vi "DAC Run.vi"(8 "error in":errorcluster, 11 "DAC Traverse in":refnum<class "DAC Traverse.lvclass">) -> (0 "error out":errorcluster, 3 "DAC Traverse out":refnum<class "DAC Traverse.lvclass">)   [LabVIEW 2019, in "DAC.lvlib" / "DAC Traverse.lvclass"]
uses:
  DAC Traverse.lvclass
  C:/Users/krio/Documents/LV_Projects/test-stand/App/DAC/DAC.lvclass
  DAC.lvclass/DAC.ctl
  Results/Results Method.ctl
  Results/Water Tunnel Results/Water Tunnel Results.lvclass
  DAC Traverse.lvclass/DAC Traverse.ctl
  DAC.lvclass
  Results/Results.lvlib
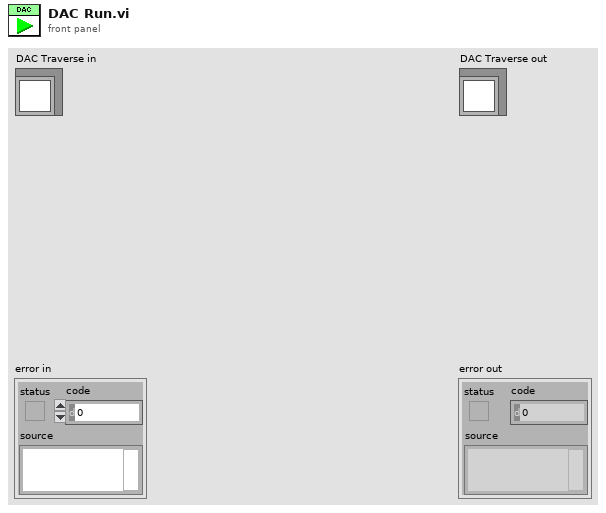
[diagram p1: front panel]
types:
  T1 = typedef "Results.lvlib/Results Method.ctl" = enum16{"Get", "Set"}
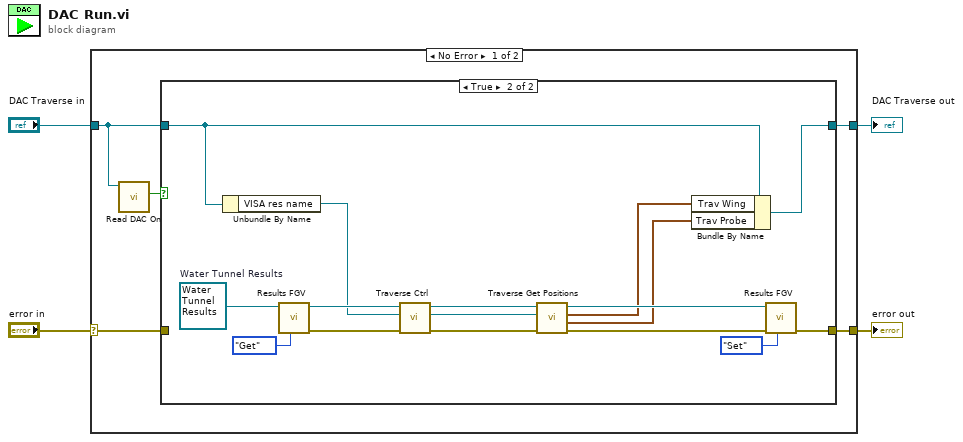
[diagram p0: block diagram]
diagram:
  n1 = case shown="No Error" "error in" {
    selector: "error in" -> [w7 w29]
    tunnel: [w6 w29] -> w2
    tunnel: [w8 w28] -> w1
    tunnel: "DAC Traverse in" -> [w5 w28]
    frame No Error {
      n2 = call "Read DAC On.vi"("DAC in"=w5) -> ("DAC On"=w9:bool)  [unwired: 8 in, 2 out]
      n3 = case shown="True" w9 {
        tunnel: w5 -> [w11 w27]
        tunnel: [w11 w24] -> w8
        tunnel: w7 -> [w10 _]
        tunnel: [w10 w23] -> w6
        frame False {
        }
        frame True {
          w22 = refnum<class "Water Tunnel Results.lvclass"> refnum  # Water Tunnel Results
          n4 = Unbundle By Name(w27) -> ("VISA res name"=w19:refnum<visa-resource-name>)
          n5 = call-dynamic "Results FGV.vi"("Method"=Results_Method."Get", "Water Tunnel Results in"=w22) -> ("error out"=w20:errorcluster, "Water Tunnel  Results out"=w21:refnum<class "Water Tunnel Results.lvclass">)  [unwired: 8 in]
          n6 = call "Traverse Ctrl.vi"("error in"=w20, "VISA resource name"=w19, "Water Tunnel Results in"=w21) -> ("error out"=w17:errorcluster, "VISA resource name out"=w12:refnum<visa-resource-name>, "Water Tunnel Results out"=w18:refnum<class "Water Tunnel Results.lvclass">)  [unwired: 6 in]
          n7 = call "Traverse Get Positions.vi"("error in"=w17, "VISA resource name"=w12, "Water Tunnel Results in"=w18) -> ("error out"=w16:errorcluster, "Trav Probe"=w13:cluster{"Px":dbl, "Py":dbl, "Pz":dbl}, "Trav Wing"=w14:cluster{"Wx":dbl, "Wy":dbl, "Wz":dbl}, "Water Tunnel Results out"=w15:refnum<class "Water Tunnel Results.lvclass">)  [unwired: 5 in]
          n8 = Bundle By Name(cluster=w27, "Trav Wing"=w14, "Trav Probe"=w13) -> (w24:refnum<class "DAC Traverse.lvclass">)
          n9 = call-dynamic "Results FGV.vi"("Method"=Results_Method."Set", "error in"=w16, "Water Tunnel Results in"=w15) -> ("error out"=w23:errorcluster)  [unwired: 7 in, 1 out]
        }
      }
    }
    frame Error {
    }
  }
  "error out" <- w2
  "DAC Traverse out" <- w1
